vi "Exercise 3.2-Data.vi"() -> ()   [LabVIEW 2012]
panel:
  out "Meter":dbl(knob) scale=0.0..2000.0
  out "Waveform Chart":dynamicdata(graph)
  in  "stop":bool
  out "Frequency":dbl
  out "Amplitude":dbl
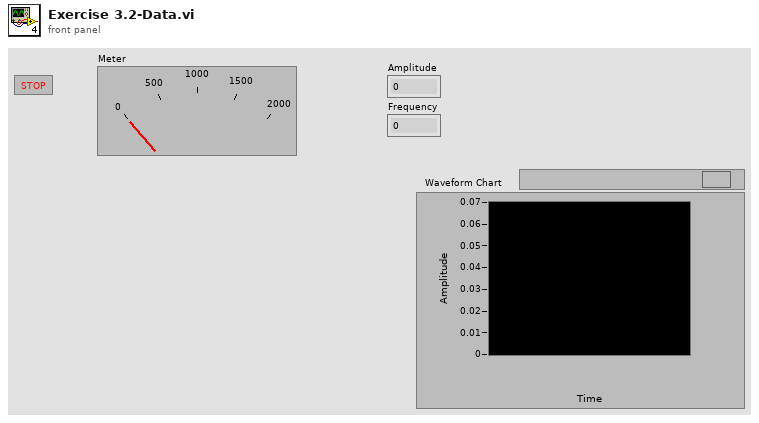
[diagram p1: front panel]
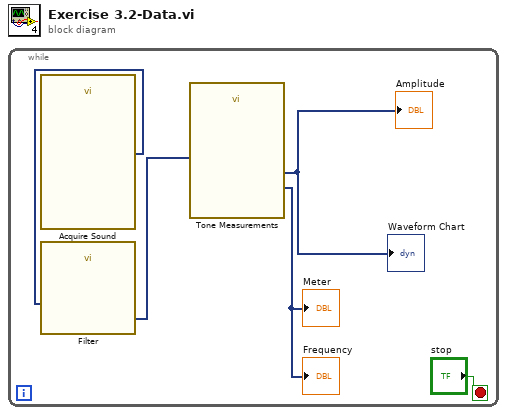
[diagram p0: block diagram]
diagram:
  n1 = while {
    stop <- "stop" stop-if-true
    n2 = call "Acquire Sound"() -> ("Data"=w3:dynamicdata)  [unwired: 18 in, 1 out]
    n3 = call "Filter"("Signal"=w3) -> ("Filtered Signal"=w2:dynamicdata)  [unwired: 9 in, 1 out]
    n4 = call "Tone Measurements"("Signals"=w2) -> ("Frequency"=→"Frequency" →"Meter":dynamicdata, "Amplitude"=→"Amplitude" →"Waveform Chart":dynamicdata)  [unwired: 8 in, 1 out]
  }
